vi "BRig_RT_panel_cue_v1,10.vi"(7 "input_setValues":bool, 11 "input_dataExp":u16[](array[numeric])) -> (3 "output_dataExp":u16[](array[numeric]))   [LabVIEW 2014]
panel:
  in  "Cue2Switch_Count_PostR":u16
  in  "Cue2Switch_Prob_PostR":u16
  in  "Cue2Switch_PostR":u16(slide) max=3 step=1 scale=0.0..3.0
  in  "Cue2Switch_Count_PreR":u16
  in  "Cue2Switch_Count_First":u16
  in  "Cue2Switch_Prob_PreR":u16
  in  "Cue2Switch_PreR":u16(slide) max=3 step=1 scale=0.0..3.0
  in  "Cue2Switch_Prob_First":u16
  in  "Cue2Switch_First":u16(slide) max=3 step=1 scale=0.0..3.0
  in  "CueLed_baseline":bool
  in  "CueSwitch_Count_PostR":u16
  in  "CueSwitch_Prob_PostR":u16
  in  "CueSwitch_PostR":u16(slide) max=3 step=1 scale=0.0..3.0
  in  "CueSwitch_Count_PreR":u16
  in  "CueSwitch_Count_First":u16
  in  "CueSwitch_Prob_PreR":u16
  in  "CueSwitch_PreR":u16(slide) max=3 step=1 scale=0.0..3.0
  in  "CueSwitch_Prob_First":u16
  in  "CueSwitch_First":u16(slide) max=3 step=1 scale=0.0..3.0
  in  "CueLed_Freq":u16=10
  in  "CueLed_Tpeak":u16=2
  in  "sp_RightSpout":u16(slide)=2 max=2 step=1 scale=0.0..2.0
  in  "sp_LeftSpout":u16(slide)=2 max=2 step=1 scale=0.0..2.0
  in  "Audio_Amp__R":u16=100 caption="Amp"
  in  "Audio_Freq__R":u16=5 caption="Freq [kHz]" max=14 step=1
  in  "Audio_Amp__L":u16=100 caption="Amp"
  in  "Audio_Freq__L":u16=5 caption="Freq [kHz]" max=14 step=1
  # "Cue State\n                                  Cue Type           LED Probability [%]      Count"
  # "Audio or LED"
  # "First"
  # "Pre Reward"
  # "Post Reward"
  # "Cue2 State\n                                  Cue Type           LED Probability [%]      Count"
  # "First"
  # "Pre Reward"
  # "Post Reward"
  # "Audio Parameters"
  # "Cue LED Parameters"
  # "Left                  Right"
  # "Frequency\n[Hz]"
  # "Frequency\n[kHz]"
  # "Timing [ms]\n                    Peak Width"
  # "Amp\n(0 - 32,000)"
  # "Speaker\nPattern\nDuring Cue"
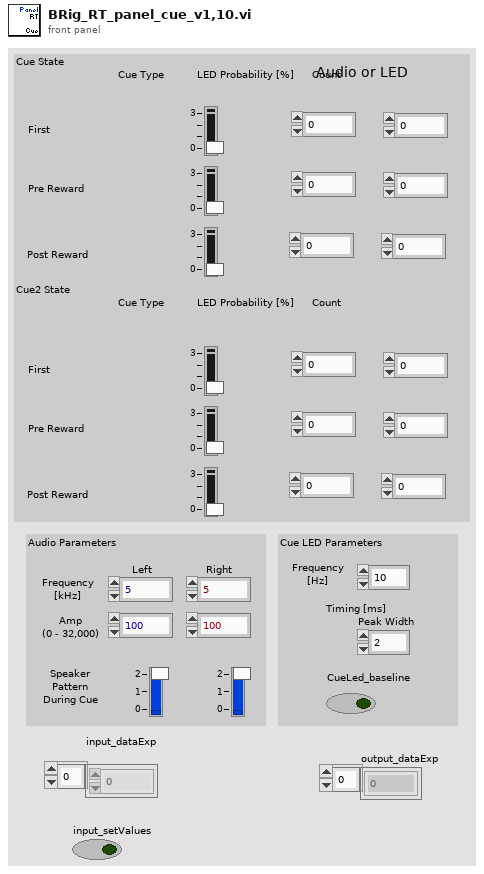
[diagram p1: front panel]
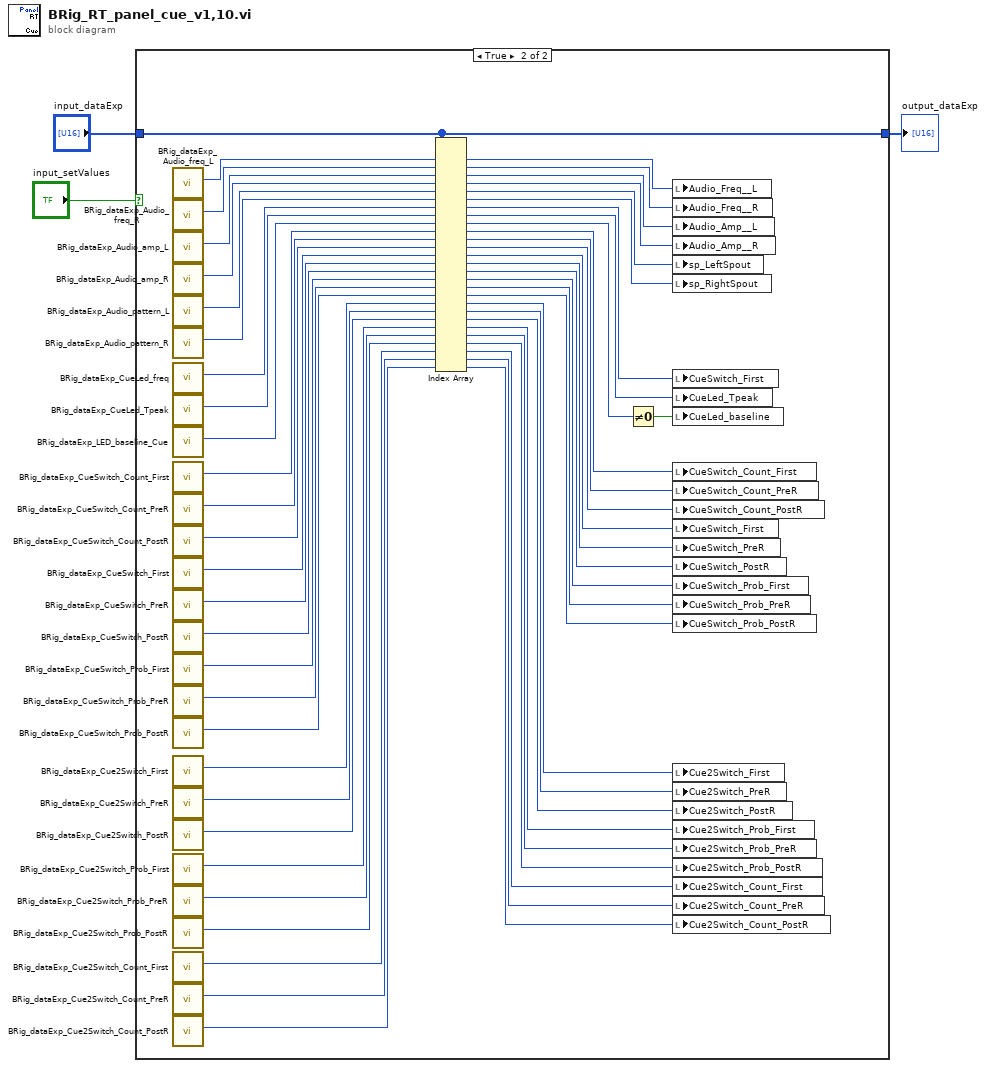
[diagram p0: block diagram]
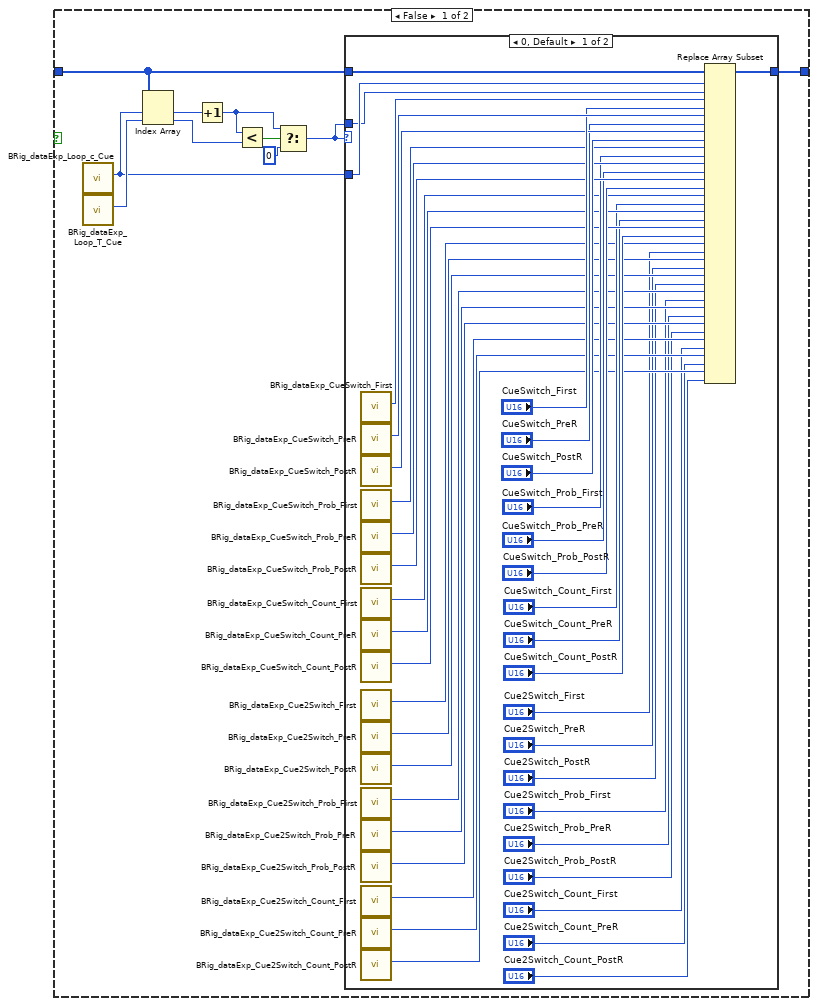
[diagram p2: hidden frame]
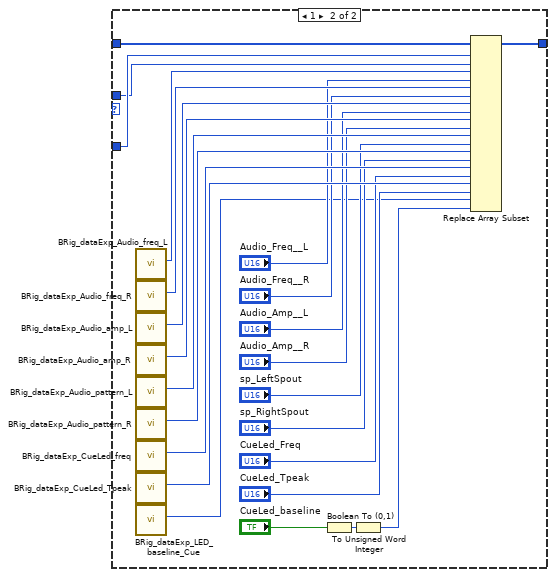
[diagram p3: hidden frame]
diagram:
  n1 = case shown="True" "input_setValues" {
    tunnel: "input_dataExp" -> [w7 w133]
    tunnel: [w6 w133] -> w2
    frame False {
      n2 = call "BRig_dataExp_Loop_c_Cue.vi"() -> ("output_Loop_c_Cue"=w5:i32)  [unwired: 11 in]
      n3 = call "BRig_dataExp_Loop_T_Cue.vi"() -> ("output_Loop_T_Cue"=w13:i32)  [unwired: 11 in]
      n4 = Index Array(array=w7, index #1=w5, index #2=w13) -> (element #1=w12:u16, element #2=w11:u16)
      n5 = Increment(x=w12) -> (x+1=w9:u16)
      n6 = Less?(x=w9, y=w11) -> (x < y?=w10:bool)
      n7 = Select(t=w9, s=w10, f=u16 0) -> (s? t:f=w4:u16)
      n8 = case shown="0, Default" w4 {
        tunnel: w7 -> [w53 w77]
        tunnel: [w34 w76] -> w6
        tunnel: w5 -> [w33 w75]
        tunnel: w4 -> [w32 w74]
        frame 0, Default {
          n9 = call "BRig_dataExp_CueSwitch_First.vi"() -> ("output_CueSwitch_First"=w52:i32)  [unwired: 11 in]
          n10 = call "BRig_dataExp_CueSwitch_PreR.vi"() -> ("output_CueSwitch_PreR"=w51:i32)  [unwired: 11 in]
          n11 = call "BRig_dataExp_CueSwitch_PostR.vi"() -> ("output_CueSwitch_PostR"=w49:i32)  [unwired: 11 in]
          n12 = call "BRig_dataExp_CueSwitch_Prob_First.vi"() -> ("output_CueSwitch_Prob_First"=w46:i32)  [unwired: 11 in]
          n13 = call "BRig_dataExp_CueSwitch_Prob_PreR.vi"() -> ("output_CueSwitch_Prob_PreR"=w45:i32)  [unwired: 11 in]
          n14 = call "BRig_dataExp_CueSwitch_Prob_PostR.vi"() -> ("output_CueSwitch_Prob_PostR"=w44:i32)  [unwired: 11 in]
          n15 = call "BRig_dataExp_CueSwitch_Count_First.vi"() -> ("output_CueSwitch_Count_First"=w40:i32)  [unwired: 11 in]
          n16 = call "BRig_dataExp_CueSwitch_Count_PreR.vi"() -> ("output_CueSwitch_Count_PreR"=w39:i32)  [unwired: 11 in]
          n17 = call "BRig_dataExp_CueSwitch_Count_PostR.vi"() -> ("output_CueSwitch_Count_PostR"=w38:i32)  [unwired: 11 in]
          n18 = call "BRig_dataExp_Cue2Switch_First.vi"() -> ("output_Cue2Switch_First"=w31:i32)  [unwired: 11 in]
          n19 = call "BRig_dataExp_Cue2Switch_PreR.vi"() -> ("output_Cue2Switch_PreR"=w30:i32)  [unwired: 11 in]
          n20 = call "BRig_dataExp_Cue2Switch_PostR.vi"() -> ("output_Cue2Switch_PostR"=w29:i32)  [unwired: 11 in]
          n21 = call "BRig_dataExp_Cue2Switch_Prob_First.vi"() -> ("output_Cue2Switch_Prob_First"=w28:i32)  [unwired: 11 in]
          n22 = call "BRig_dataExp_Cue2Switch_Prob_PreR.vi"() -> ("output_Cue2Switch_Prob_PreR"=w27:i32)  [unwired: 11 in]
          n23 = call "BRig_dataExp_Cue2Switch_Prob_PostR.vi"() -> ("output_Cue2Switch_Prob_PostR"=w26:i32)  [unwired: 11 in]
          n24 = call "BRig_dataExp_Cue2Switch_Count_First.vi"() -> ("output_Cue2Switch_Count_First"=w25:i32)  [unwired: 11 in]
          n25 = call "BRig_dataExp_Cue2Switch_Count_PreR.vi"() -> ("output_Cue2Switch_Count_PreR"=w24:i32)  [unwired: 11 in]
          n26 = call "BRig_dataExp_Cue2Switch_Count_PostR.vi"() -> ("output_Cue2Switch_Count_PostR"=w23:i32)  [unwired: 11 in]
          n27 = Replace Array Subset(array=w53, new element #1=w32, index #1=w33, new element #2="CueSwitch_First", index #2=w52, new element #3="CueSwitch_PreR", index #3=w51, new element #4="CueSwitch_PostR", index #4=w49, new element #5="CueSwitch_Prob_First", index #5=w46, new element #6="CueSwitch_Prob_PreR", index #6=w45, new element #7="CueSwitch_Prob_PostR", index #7=w44, new element #8="CueSwitch_Count_First", index #8=w40, new element #9="CueSwitch_Count_PreR", index #9=w39, new element #10="CueSwitch_Count_PostR", index #10=w38, new element #11="Cue2Switch_First", index #11=w31, new element #12="Cue2Switch_PreR", index #12=w30, new element #13="Cue2Switch_PostR", index #13=w29, new element #14="Cue2Switch_Prob_First", index #14=w28, new element #15="Cue2Switch_Prob_PreR", index #15=w27, new element #16="Cue2Switch_Prob_PostR", index #16=w26, new element #17="Cue2Switch_Count_First", index #17=w25, new element #18="Cue2Switch_Count_PreR", index #18=w24, new element #19="Cue2Switch_Count_PostR", index #19=w23) -> (w34:u16[])
        }
        frame 1 {
          n28 = call "BRig_dataExp_Audio_freq_L.vi"() -> ("output_Audio_freq__L"=w73:i32)  [unwired: 11 in]
          n29 = call "BRig_dataExp_Audio_freq_R.vi"() -> ("output_Audio_freq__R"=w72:i32)  [unwired: 11 in]
          n30 = call "BRig_dataExp_Audio_amp_L.vi"() -> ("output_Audio_amp__L"=w71:i32)  [unwired: 11 in]
          n31 = call "BRig_dataExp_Audio_amp_R.vi"() -> ("output_Audio_amp__R"=w70:i32)  [unwired: 11 in]
          n32 = call "BRig_dataExp_Audio_pattern_L.vi"() -> ("output_Audio_sp__L"=w69:i32)  [unwired: 11 in]
          n33 = call "BRig_dataExp_Audio_pattern_R.vi"() -> ("output_Audio_sp__R"=w68:i32)  [unwired: 11 in]
          n34 = call "BRig_dataExp_CueLed_freq.vi"() -> ("output_CueLed_Freq"=w67:i32)  [unwired: 11 in]
          n35 = call "BRig_dataExp_CueLed_Tpeak.vi"() -> ("output_CueLed_Tpeak"=w66:i32)  [unwired: 11 in]
          n36 = call "BRig_dataExp_LED_baseline_Cue.vi"() -> ("output_LED_baseline_Cue"=w57:i32)  [unwired: 11 in]
          n37 = Boolean To (0,1)(Boolean="CueLed_baseline") -> (0, 1=w55:i16)
          n38 = To Unsigned Word Integer(number=w55) -> (unsigned 16bit integer=w54:u16)
          n39 = Replace Array Subset(array=w77, new element #1=w74, index #1=w75, new element #2="Audio_Freq__L", index #2=w73, new element #3="Audio_Freq__R", index #3=w72, new element #4="Audio_Amp__L", index #4=w71, new element #5="Audio_Amp__R", index #5=w70, new element #6="sp_LeftSpout", index #6=w69, new element #7="sp_RightSpout", index #7=w68, new element #8="CueLed_Freq", index #8=w67, new element #9="CueLed_Tpeak", index #9=w66, new element #10=w54, index #10=w57) -> (w76:u16[])
        }
      }
    }
    frame True {
      n40 = call "BRig_dataExp_Audio_freq_L.vi"() -> ("output_Audio_freq__L"=w132:i32)  [unwired: 11 in]
      n41 = call "BRig_dataExp_Audio_freq_R.vi"() -> ("output_Audio_freq__R"=w130:i32)  [unwired: 11 in]
      n42 = call "BRig_dataExp_Audio_amp_L.vi"() -> ("output_Audio_amp__L"=w128:i32)  [unwired: 11 in]
      n43 = call "BRig_dataExp_Audio_amp_R.vi"() -> ("output_Audio_amp__R"=w126:i32)  [unwired: 11 in]
      n44 = call "BRig_dataExp_Audio_pattern_L.vi"() -> ("output_Audio_sp__L"=w124:i32)  [unwired: 11 in]
      n45 = call "BRig_dataExp_Audio_pattern_R.vi"() -> ("output_Audio_sp__R"=w123:i32)  [unwired: 11 in]
      n46 = call "BRig_dataExp_CueLed_freq.vi"() -> ("output_CueLed_Freq"=w120:i32)  [unwired: 11 in]
      n47 = call "BRig_dataExp_CueLed_Tpeak.vi"() -> ("output_CueLed_Tpeak"=w118:i32)  [unwired: 11 in]
      n48 = call "BRig_dataExp_LED_baseline_Cue.vi"() -> ("output_LED_baseline_Cue"=w116:i32)  [unwired: 11 in]
      n49 = call "BRig_dataExp_CueSwitch_Count_First.vi"() -> ("output_CueSwitch_Count_First"=w113:i32)  [unwired: 11 in]
      n50 = call "BRig_dataExp_CueSwitch_Count_PreR.vi"() -> ("output_CueSwitch_Count_PreR"=w112:i32)  [unwired: 11 in]
      n51 = call "BRig_dataExp_CueSwitch_Count_PostR.vi"() -> ("output_CueSwitch_Count_PostR"=w111:i32)  [unwired: 11 in]
      n52 = call "BRig_dataExp_CueSwitch_First.vi"() -> ("output_CueSwitch_First"=w110:i32)  [unwired: 11 in]
      n53 = call "BRig_dataExp_CueSwitch_PreR.vi"() -> ("output_CueSwitch_PreR"=w109:i32)  [unwired: 11 in]
      n54 = call "BRig_dataExp_CueSwitch_PostR.vi"() -> ("output_CueSwitch_PostR"=w108:i32)  [unwired: 11 in]
      n55 = call "BRig_dataExp_CueSwitch_Prob_First.vi"() -> ("output_CueSwitch_Prob_First"=w107:i32)  [unwired: 11 in]
      n56 = call "BRig_dataExp_CueSwitch_Prob_PreR.vi"() -> ("output_CueSwitch_Prob_PreR"=w106:i32)  [unwired: 11 in]
      n57 = call "BRig_dataExp_CueSwitch_Prob_PostR.vi"() -> ("output_CueSwitch_Prob_PostR"=w105:i32)  [unwired: 11 in]
      n58 = call "BRig_dataExp_Cue2Switch_First.vi"() -> ("output_Cue2Switch_First"=w95:i32)  [unwired: 11 in]
      n59 = call "BRig_dataExp_Cue2Switch_PreR.vi"() -> ("output_Cue2Switch_PreR"=w94:i32)  [unwired: 11 in]
      n60 = call "BRig_dataExp_Cue2Switch_PostR.vi"() -> ("output_Cue2Switch_PostR"=w93:i32)  [unwired: 11 in]
      n61 = call "BRig_dataExp_Cue2Switch_Prob_First.vi"() -> ("output_Cue2Switch_Prob_First"=w92:i32)  [unwired: 11 in]
      n62 = call "BRig_dataExp_Cue2Switch_Prob_PreR.vi"() -> ("output_Cue2Switch_Prob_PreR"=w91:i32)  [unwired: 11 in]
      n63 = call "BRig_dataExp_Cue2Switch_Prob_PostR.vi"() -> ("output_Cue2Switch_Prob_PostR"=w90:i32)  [unwired: 11 in]
      n64 = call "BRig_dataExp_Cue2Switch_Count_First.vi"() -> ("output_Cue2Switch_Count_First"=w89:i32)  [unwired: 11 in]
      n65 = call "BRig_dataExp_Cue2Switch_Count_PreR.vi"() -> ("output_Cue2Switch_Count_PreR"=w88:i32)  [unwired: 11 in]
      n66 = call "BRig_dataExp_Cue2Switch_Count_PostR.vi"() -> ("output_Cue2Switch_Count_PostR"=w87:i32)  [unwired: 11 in]
      n67 = Index Array(array=w133, index #1=w132, index #2=w130, index #3=w128, index #4=w126, index #5=w124, index #6=w123, index #7=w120, index #8=w118, index #9=w116, index #10=w113, index #11=w112, index #12=w111, index #13=w110, index #14=w109, index #15=w108, index #16=w107, index #17=w106, index #18=w105, index #19=w95, index #20=w94, index #21=w93, index #22=w92, index #23=w91, index #24=w90, index #25=w89, index #26=w88, index #27=w87) -> (element #1=w131:u16, element #2=w129:u16, element #3=w127:u16, element #4=w125:u16, element #5=w122:u16, element #6=w121:u16, element #7=w119:u16, element #8=w117:u16, element #9=w114:u16, element #10=w104:u16, element #11=w103:u16, element #12=w102:u16, element #13=w101:u16, element #14=w100:u16, element #15=w99:u16, element #16=w98:u16, element #17=w97:u16, element #18=w96:u16, element #19=w86:u16, element #20=w85:u16, element #21=w84:u16, element #22=w83:u16, element #23=w82:u16, element #24=w81:u16, element #25=w80:u16, element #26=w79:u16, element #27=w78:u16)
      n68 = Not Equal To 0?(x=w114) -> (x != 0?=w115:bool)
      n69 = local write "Audio_Freq__L"(w131) -> ()
      n70 = local write "Audio_Freq__R"(w129) -> ()
      n71 = local write "Audio_Amp__L"(w127) -> ()
      n72 = local write "Audio_Amp__R"(w125) -> ()
      n73 = local write "sp_LeftSpout"(w122) -> ()
      n74 = local write "sp_RightSpout"(w121) -> ()
      n75 = local write "CueSwitch_First"(w119) -> ()
      n76 = local write "CueLed_Tpeak"(w117) -> ()
      n77 = local write "CueLed_baseline"(w115) -> ()
      n78 = local write "CueSwitch_Count_First"(w104) -> ()
      n79 = local write "CueSwitch_Count_PreR"(w103) -> ()
      n80 = local write "CueSwitch_Count_PostR"(w102) -> ()
      n81 = local write "CueSwitch_First"(w101) -> ()
      n82 = local write "CueSwitch_PreR"(w100) -> ()
      n83 = local write "CueSwitch_PostR"(w99) -> ()
      n84 = local write "CueSwitch_Prob_First"(w98) -> ()
      n85 = local write "CueSwitch_Prob_PreR"(w97) -> ()
      n86 = local write "CueSwitch_Prob_PostR"(w96) -> ()
      n87 = local write "Cue2Switch_First"(w86) -> ()
      n88 = local write "Cue2Switch_PreR"(w85) -> ()
      n89 = local write "Cue2Switch_PostR"(w84) -> ()
      n90 = local write "Cue2Switch_Prob_First"(w83) -> ()
      n91 = local write "Cue2Switch_Prob_PreR"(w82) -> ()
      n92 = local write "Cue2Switch_Prob_PostR"(w81) -> ()
      n93 = local write "Cue2Switch_Count_First"(w80) -> ()
      n94 = local write "Cue2Switch_Count_PreR"(w79) -> ()
      n95 = local write "Cue2Switch_Count_PostR"(w78) -> ()
    }
  }
  "output_dataExp" <- w2
